vi "STM Write Meta.vi"(8 "error in":errorcluster, 10 "Meta data":T1[](array[typedef]), 11 "connection ID":refnum<k5>) -> (0 "error out":errorcluster, 3 "connection ID out":refnum<k5>)   [LabVIEW 2010]
doc: "Use this VI to transmit the Meta data cluster to a remote computer. Sending the meta data to another computers helps maintainability since the data resides only on one side and it is shared to other computers at run time.\n\nThe meta data cluster must contain valid name and type information before being sent.\n\nThis VI converts the meta data cluster into XML format before transfering it to a remote computer. If your application communicates with a non-LabVIEW program, you can still use this VI but make sure the receiving code knows how to parse through the XML string.\n\nCopyright 2015, 2016, 2017 National Instruments Corporation\n\nLicensed under the Apache License, Version 2.0 (the \"License\"); you may not use this file except in compliance with the License.\n\n You may obtain a copy of the License at\n\n http://www.apache.org/licenses/LICENSE-2.0\n\nUnless required by applicable law or agreed to in writing, software distributed under the License is distributed on an \"AS IS\" BASIS, WITHOUT WARRANTIES OR CONDITIONS OF ANY KIND, either express or implied.\n\nSee the License for the specific language governing permissions and limitations under the License."
uses:
  stm_MetaElement.ctl
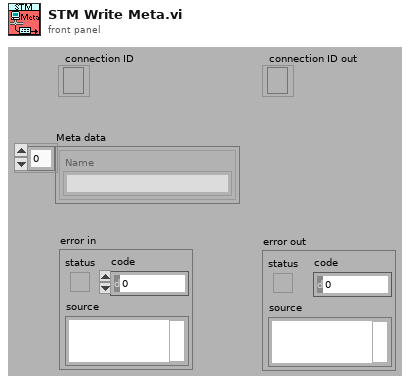
[diagram p1: front panel]
types:
  T1 = typedef "stm_MetaElement.ctl" = cluster{"Name":string}
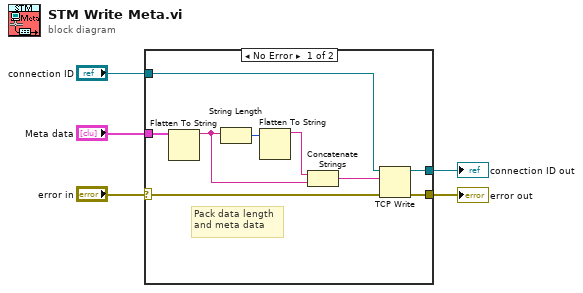
[diagram p0: block diagram]
diagram:
  n1 = case shown="No Error" "error in" {
    selector: "error in" -> [w10 w16]
    tunnel: [w14 w15] -> w5
    tunnel: "connection ID" -> [w13 w15]
    tunnel: "Meta data" -> [w12 _]
    tunnel: [w11 w16] -> w2
    frame No Error {
      # "Pack data length\nand meta data"
      n2 = Flatten To String(anything=w12) -> (data string=w6:string)  [unwired: 1 in, 4 out]
      n3 = String Length(string=w6) -> (length=w9:i32)
      n4 = Flatten To String(anything=w9) -> (data string=w8:string)  [unwired: 1 in, 4 out]
      n5 = Concatenate Strings(w8, w6) -> (w7:string)
      n6 = TCP Write(connection ID=w13, data in=w7, error in (no error)=w10) -> (connection ID out=w14:refnum<k5>, error out=w11:errorcluster)  [unwired: 2 out]
    }
    frame Error {
    }
  }
  "connection ID out" <- w5
  "error out" <- w2
